vi "FakeGlobals.vi"() -> ()   [LabVIEW 2021]
uses:
  <vilib>/Analysis/1siggen.llb/Ramp Pattern by Samples.vi
  <vilib>/Analysis/NI_AALBase.lvlib
panel:
  out "Mag":dbl
  out "Temp":dbl
  in  "stop":bool
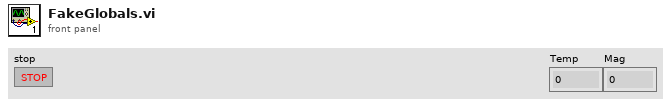
[diagram p1: front panel]
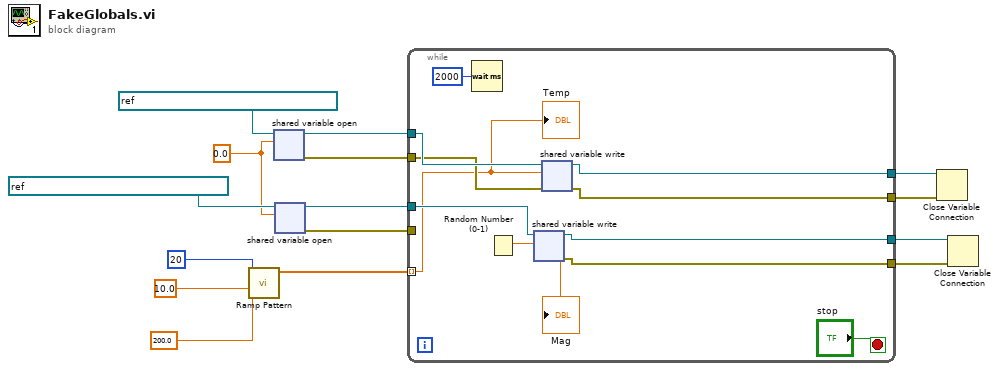
[diagram p0: block diagram]
diagram:
  w1 = 0.0
  n1 = call-poly <vilib>:"Ramp Pattern.vi"("start"=10.0, "end"=200.0, "samples"=20) -> ("Ramp Pattern"=w4:dbl[])  [unwired: 7 in, 1 out]
  n2 = shared-variable-open(refnum<k21> "ni.var.psp://localhost/FakeGlobals/T" ("shared variable refnum in"), w1) -> (w13:refnum<k21>, w10:errorcluster)  [unwired: 2 in]
  n3 = shared-variable-open(refnum<k21> "ni.var.psp://localhost/FakeGlobals/B" ("shared variable refnum in"), w1) -> (w12:refnum<k21>, w11:errorcluster)  [unwired: 2 in]
  n4 = while {
    tunnel: w13 -> [w21]
    tunnel: w12 -> [w25]
    tunnel: w11 -> [_]
    tunnel: w10 -> [w20]
    tunnel: [w23] -> w9
    tunnel: [w22] -> w8
    tunnel: w4 -> [w19] mode=indexing
    tunnel: [w18] -> w3
    tunnel: [w17] -> w2
    stop <- "stop" stop-if-true
    n5 = Wait (ms)(milliseconds to wait=u32 2000) -> ()  [unwired: 1 out]
    n6 = Random Number (0-1)() -> (number: 0 to 1=w24:dbl)
    "Mag" <- w24
    n7 = shared-variable-write(w25, w24) -> (w22:refnum<k21>, w23:errorcluster)  [unwired: 1 in]
    n8 = shared-variable-write(w21, w20, w19) -> (w18:refnum<k21>, w17:errorcluster)
    "Temp" <- w19
  }
  n9 = Close Variable Connection(8:w2, 11:w3) -> ()  [unwired: 1 out]
  n10 = Close Variable Connection(8:w9, 11:w8) -> ()  [unwired: 1 out]
